vi "EEPROM Tester Info.vi"() -> (0 "EEPROM Tester Info":T1)   [LabVIEW 2010, in "lib1299.lvlib"]
uses:
  lib1299.lvlib
  Controls/EEPROM Tester Info.ctl
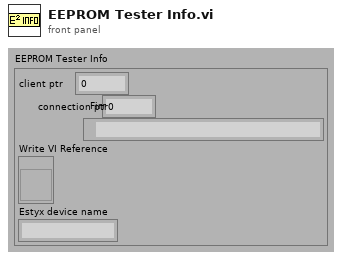
[diagram p1: front panel]
types:
  T1 = typedef "lib1299.lvlib/EEPROM Tester Info.ctl" = cluster{"client ptr":u32, "connection ptr":u32, "Firmware file":path, "Write VI Reference":refnum<vi>, "Estyx device name":string}
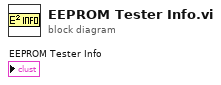
[diagram p0: block diagram]
diagram:
